vi "19.7-ClassicIIR-Type-CompareH(w).vi"() -> ()   [LabVIEW 2020]
doc: "Displays the Transfer Function of the filter selected from the front panel controls. \n\nYou can select any of the 5 IIR filter design methods (Bessel, Butterworth, Chebyshev I and II, and Elliptic) and the passband type (lowpass, highpass, bandpass, and bandstop)."
uses:
  <vilib>/Analysis/3filter.llb/Filter Passband Type.ctl
  <vilib>/Analysis/NI_AALPro.lvlib
  <vilib>/Analysis/NI_AALBase.lvlib
panel:
  in  "Order":i32(slide)=6 scale=1.0..20.0
  out "Phase":cluster{dbl, dbl, dbl[]}[](graph)
  in  "LowCutoff(3dB)":dbl=250.0 format="%#.6g"
  in  "HighCutoff(3dB)":dbl=450.0 format="%#.6g"
  out "Mag":cluster{dbl, dbl, dbl[]}[](graph)
  in  "Type":T1
  in  "Stop":bool
  in  "Fs":dbl=1024.0 format="%#.6g"
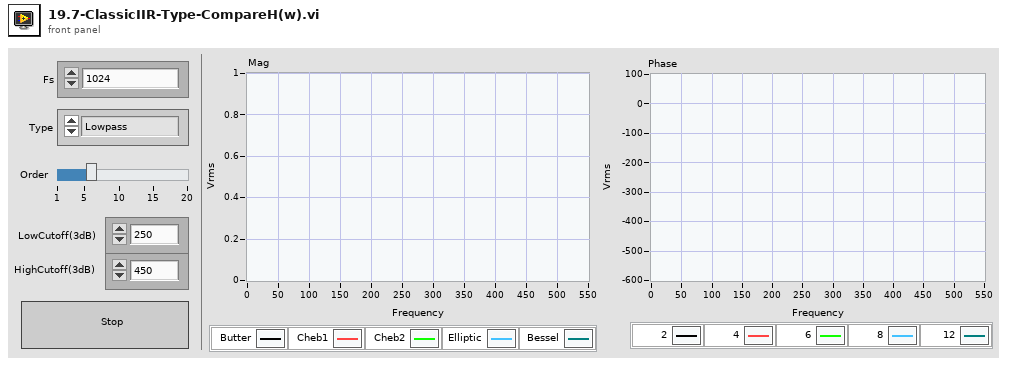
[diagram p1: front panel]
types:
  T1 = typedef "NI_AALBase.lvlib/Filter Passband Type.ctl" = enum32{"Lowpass", "Highpass", "Bandpass", "Bandstop"}
  T2 = enum32{"Vrms", "Vpk", "Vrms^2", "Vpk^2", "Vrms/rtHz", "Vpk/rtHz", "Vrms^2/Hz", "Vpk^2/Hz"}
  T3 = enum16{"Power (Vrms^2)", "Amplitude (Vrms)", "Gain (amplitude ratio)"}
  T4 = cluster{"filter structure":enum32{"IIR 2nd Order", "IIR 4th Order"}, "Reverse Coefficients":dbl[], "Forward Coefficients":dbl[]}
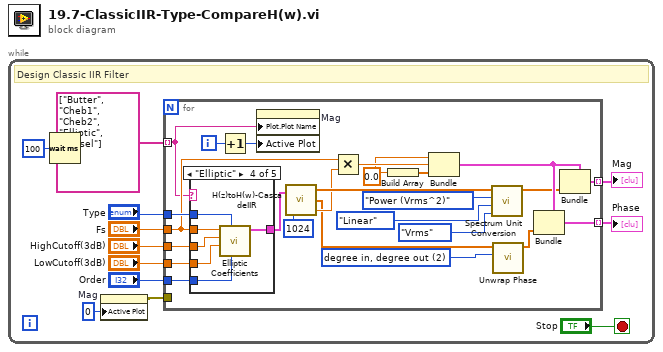
[diagram p0: block diagram]
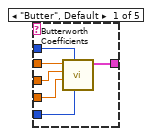
[diagram p2: hidden frame]
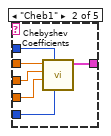
[diagram p3: hidden frame]
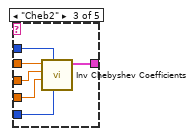
[diagram p4: hidden frame]
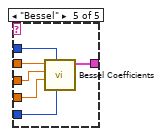
[diagram p5: hidden frame]
diagram:
  n1 = while {
    stop <- "Stop" stop-if-true
    # "Design Classic IIR Filter"
    n2 = Wait (ms)(milliseconds to wait=u32 100) -> ()  [unwired: 1 out]
    n3 = property on="Mag" class="WFGraph (strict)"("Active Plot"=u32 0) -> (error out=w1:errorcluster)  [unwired: 2 in, 1 out]
    n4 = for {
      tunnel: "Type" -> [w37]
      tunnel: "Fs" -> [w36]
      tunnel: [w35] -> w8 mode=indexing
      tunnel: "HighCutoff(3dB)" -> [w34]
      tunnel: "LowCutoff(3dB)" -> [w33]
      tunnel: [w32] -> w4 mode=indexing
      tunnel: string[] ["Butter", "Cheb1", "Cheb2", "Elliptic", "Bessel"] -> [w13] mode=indexing
      tunnel: "Order" -> [w16]
      tunnel: w1 -> [_]
      i -> [w14]
      w22 = 0.0
      w26 = 2 items=["radian in, radian out", "radian in, degree out", "degree in, degree out", "degree in, radian out"] ("phase unit")
      n5 = case shown="\"Elliptic\"" w13 {
        tunnel: w37 -> [w41 w48 w55 w61 w66]
        tunnel: w36 -> [w42 w47 w53 w59 w65]
        tunnel: [w43 w49 w54 w60 w67] -> w21
        tunnel: w34 -> [w40 w46 w52 w58 w63]
        tunnel: w33 -> [w39 w45 w51 w57 w64]
        tunnel: w16 -> [w38 w44 w50 w56 w62]
        frame "Butter", Default {
          n6 = call <vilib>:"Butterworth Coefficients.vi"("order"=w38, "filter type"=w41, "low cutoff freq: fl"=w39, "high cutoff freq: fh"=w40, "sampling freq: fs"=w42) -> ("IIR Filter Cluster"=w43:T4)  [unwired: 5 in, 1 out]
        }
        frame "Cheb1" {
          n7 = call <vilib>:"Chebyshev Coefficients.vi"("order"=w44, "filter type"=w48, "low cutoff freq: fl"=w45, "high cutoff freq: fh"=w46, "sampling freq: fs"=w47) -> ("IIR Filter Cluster"=w49:T4)  [unwired: 5 in, 1 out]
        }
        frame "Cheb2" {
          n8 = call <vilib>:"Inv Chebyshev Coefficients.vi"("order"=w50, "filter type"=w55, "low cutoff freq: fl"=w51, "high cutoff freq: fh"=w52, "sampling freq: fs"=w53) -> ("IIR Filter Cluster"=w54:T4)  [unwired: 5 in, 1 out]
        }
        frame "Elliptic" {
          n9 = call <vilib>:"Elliptic Coefficients.vi"("order"=w56, "filter type"=w61, "low cutoff freq: fl"=w57, "high cutoff freq: fh"=w58, "sampling freq: fs"=w59) -> ("IIR Filter Cluster"=w60:T4)  [unwired: 5 in, 1 out]
        }
        frame "Bessel" {
          n10 = call <vilib>:"Bessel Coefficients.vi"("order"=w62, "filter type"=w66, "low cutoff freq: fl"=w64, "high cutoff freq: fh"=w63, "sampling freq: fs"=w65) -> ("IIR Filter Cluster"=w67:T4)  [unwired: 5 in, 1 out]
        }
      }
      n11 = Increment(x=w14) -> (x+1=w15:i32)
      n12 = property on="Mag" class="WFGraph (strict)"("Plot.Plot Name"=w13, "Active Plot"=w15) -> ()  [unwired: 2 in, 2 out]
      n13 = call "H(z)toH(w)-CascadeIIR.vi"("IIR Filter Cluster"=w21, "FFT size"=1024) -> ("Mag H(w)"=w20:dbl[], "Phase H(w)"=w18:dbl[], "df"=w19:dbl)
      n14 = Multiply(x=w36, y=w19) -> (x*y=w29:dbl)
      n15 = Build Array ("array")(w22) -> (w28:dbl[])
      n16 = Bundle(w22, w29, w28) -> (w31:cluster{dbl, dbl, dbl[]})  [unwired: 1 in]
      n17 = call <vilib>:"Spectrum Unit Conversion.vi"("display unit"=T2."Vrms", "log/linear"=enum16{"Linear", "dB", "dBm"}."Linear", "spectrum type"=T3."Power (Vrms^2)", "Spectrum in"=w20) -> ("Spectrum out"=w27:dbl[])  [unwired: 6 in, 1 out]
      n18 = call <vilib>:"Unwrap Phase.vi"("phase unit"=w26, "Phase"=w18) -> ("Unwrapped Phase"=w30:dbl[])  [unwired: 8 in, 1 out]
      n19 = Bundle(cluster=w31, w30) -> (w32:cluster{dbl, dbl, dbl[]})  [unwired: 2 in]
      n20 = Bundle(cluster=w31, w27) -> (w35:cluster{dbl, dbl, dbl[]})  [unwired: 2 in]
    }
    "Mag" <- w8
    "Phase" <- w4
  }
